vi "interpolate_path.vi"(8 "error in (no error)":errorcluster, 11 "Position Array":cluster{"X":i32, "Y":i32}[](array[cluster])) -> (0 "error out":errorcluster, 3 "Interploated points":dbl[][](array[numeric]))   [LabVIEW 2011]
uses:
  <vilib>/gmath/NI_Gmath.lvlib
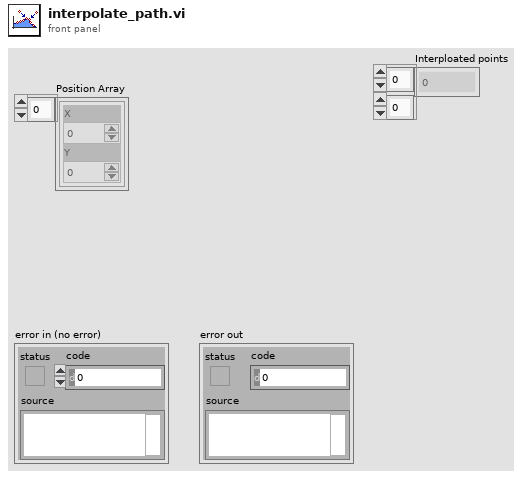
[diagram p1: front panel]
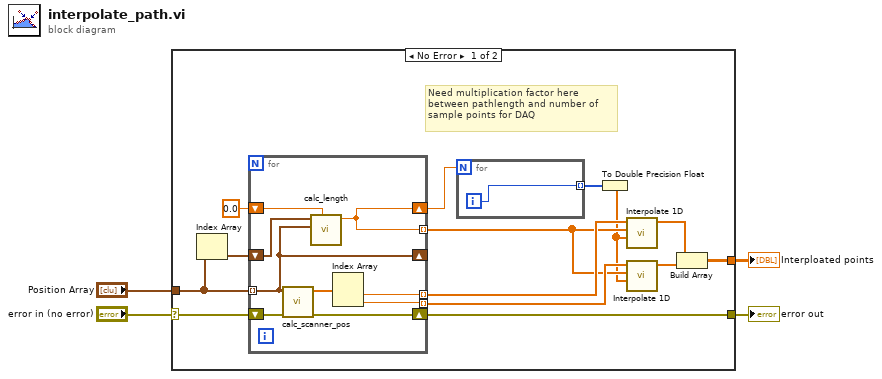
[diagram p0: block diagram]
diagram:
  n1 = case shown="No Error" "error in (no error)" {
    selector: "error in (no error)" -> [w7 w29]
    tunnel: [w18 w29] -> w4
    tunnel: "Position Array" -> [w17 _]
    tunnel: [w8 _] -> w2
    frame No Error {
      # "Need multiplication factor here\nbetween pathlength and number of\nsample points for DAQ"
      n2 = Index Array(array=w17) -> (element=w16:cluster{"X":i32, "Y":i32})  [unwired: 1 in]
      n3 = for {
        tunnel: w17 -> [w23] mode=indexing
        tunnel: [w25] -> w14 mode=indexing
        tunnel: [w24] -> w13 mode=indexing
        shift-right: [w27] -> w18
        shift-left: w7 -> [w28]
        shift-right: [w23] -> _
        shift-left: w16 -> [w22]
        shift-right: [w20] -> w11
        shift-left: 0.0 ("New length") -> [w21]
        tunnel: [w20] -> w12 mode=indexing
        n4 = call "calc_scanner_pos.vi"("error in (no error)"=w28, "Mouse position"=w23) -> ("error out"=w27:errorcluster, "Scanner position"=w26:dbl[])  [unwired: 8 in]
        n5 = call "calc_length.vi"("Old length"=w21, "Current point"=w23, "Last point"=w22) -> ("New length"=w20:dbl)  [unwired: 8 in]
        n6 = Index Array(array=w26) -> (element #1=w25:dbl, element #2=w24:dbl)  [unwired: 2 in]
      }
      n7 = for {
        N: w11 -> [_]
        tunnel: [w19] -> w6 mode=indexing
        i -> [w19]
      }
      n8 = To Double Precision Float(number=w6) -> (double precision float=w5:dbl[])
      n9 = call <vilib>:"Interpolate 1D.vi"("xi"=w5, "X"=w12, "Y"=w14) -> ("yi"=w10:dbl[])  [unwired: 6 in, 2 out]
      n10 = call <vilib>:"Interpolate 1D.vi"("xi"=w5, "X"=w12, "Y"=w13) -> ("yi"=w9:dbl[])  [unwired: 6 in, 2 out]
      n11 = Build Array(w10, w9) -> (w8:dbl[][])
    }
    frame Error {
    }
  }
  "error out" <- w4
  "Interploated points" <- w2
